vi "表格清空.vi"(11 "表格控件":string[][](table)) -> (3 "表格控件out":string[][](table))   [LabVIEW 2017]
panel:
  out "大小":i32[](array[numeric])
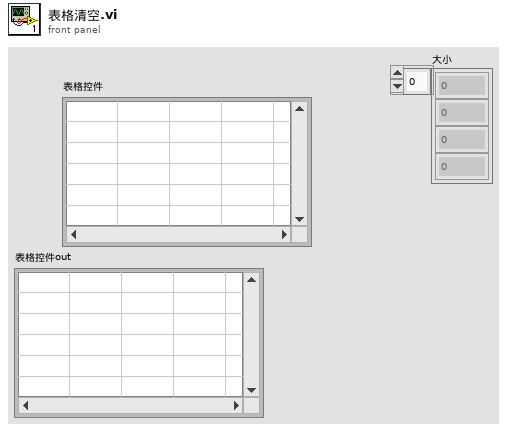
[diagram p1: front panel]
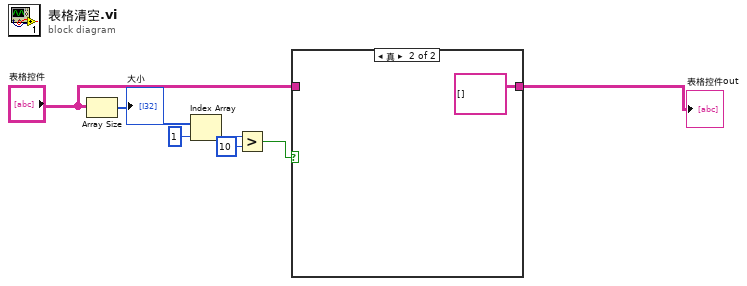
[diagram p0: block diagram]
diagram:
  n1 = Array Size(array="表格控件") -> (size(s)=w7:i32[])
  "大小" <- w7
  n2 = Index Array(array=w7, index=1 ("索引")) -> (element=w5:i32)
  n3 = Greater?(x=w5, y=10) -> (0:w3:bool)
  n4 = case shown="真" w3 {
    tunnel: "表格控件" -> [w8 _]
    tunnel: [w8 string[][] [] ("表格控件")] -> w1
    frame False {
    }
    frame True {
    }
  }
  "表格控件out" <- w1
